vi "4bit Binary.vi"() -> ()   [LabVIEW 2021]
panel:
  in  "?":bool
  out "1":bool
  out "2":bool
  out "3":bool
  out "4":bool
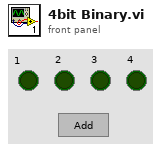
[diagram p1: front panel]
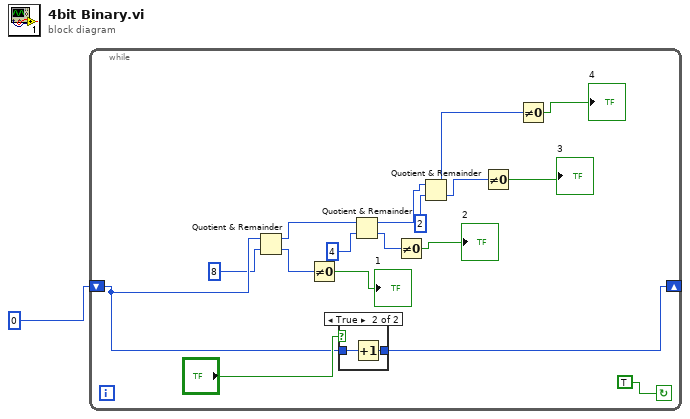
[diagram p0: block diagram]
diagram:
  n1 = while {
    shift-right: [w18] -> _
    shift-left: u16 0 -> [w16]
    stop <- TRUE continue-if-true
    n2 = Quotient & Remainder(x=w16, y=8) -> (x-y*floor(x/y)=w12:i32, floor(x/y)=w14:i32)
    n3 = Not Equal To 0?(x=w14) -> (x != 0?=→"1":bool)
    n4 = case shown="True" "?" {
      tunnel: w16 -> [w19 w21]
      tunnel: [w19 w20] -> w18
      frame False {
      }
      frame True {
        n5 = Increment(x=w21) -> (x+1=w20:u16)
      }
    }
    n6 = Quotient & Remainder(x=w12, y=4) -> (x-y*floor(x/y)=w8:i32, floor(x/y)=w10:i32)
    n7 = Not Equal To 0?(x=w10) -> (x != 0?=→"2":bool)
    n8 = Quotient & Remainder(x=w8, y=2) -> (x-y*floor(x/y)=w4:i32, floor(x/y)=w6:i32)
    n9 = Not Equal To 0?(x=w6) -> (x != 0?=→"3":bool)
    n10 = Not Equal To 0?(x=w4) -> (x != 0?=→"4":bool)
  }
